vi "Startup.vi"(7 "Application in":refnum<class "Application.lvclass">, 8 "error in (no error)":errorcluster, 11 "Config in":refnum<class "Config.lvclass">) -> (0 "error out":errorcluster, 3 "Config out":refnum<class "Config.lvclass">, 5 "Application out":refnum<class "Application.lvclass">)   [LabVIEW 2019, in "Config.lvclass"]
doc: "Developed by Kevin Thompson\nkevin@thompsonengineering.net\n\nCopyright 2018-2020\nThompson Engineering, LLC"
uses:
  Config.lvclass
  Application/Application.lvclass
  DataTypes/Config Settings.ctl
  Application/DataTypes/Settings--cluster.ctl
  Main/DataTypes/Settings--cluster.ctl
  Main/support/Data Algorithms/subvis/DataTypes/Gain control.ctl
  Main/support/Data Algorithms/subvis/DataTypes/ESR scaling--cluster.ctl
  DAQ_Engine/DataTypes/Settings--cluster.ctl
  Common/DataTypes/Measurement Config--cluster.ctl
  Common/DataTypes/Acquisition Mode--cluster.ctl
  Log_Engine/DataTypes/Settings--cluster.ctl
  Config.lvclass/Config.ctl
  Application/Application.lvclass/Application.ctl
  Accessors/Get Application Settings.vi
  Application/Accessors/Set Settings.vi
  Common/Startup/GBL System.vi
  Log_Engine/Log_Engine.lvclass
  DAQ_Engine/DAQ_Engine.lvclass
  Main/Main.lvclass
  Common/DataTypes/TD GetSet ActionSelect--enum.ctl
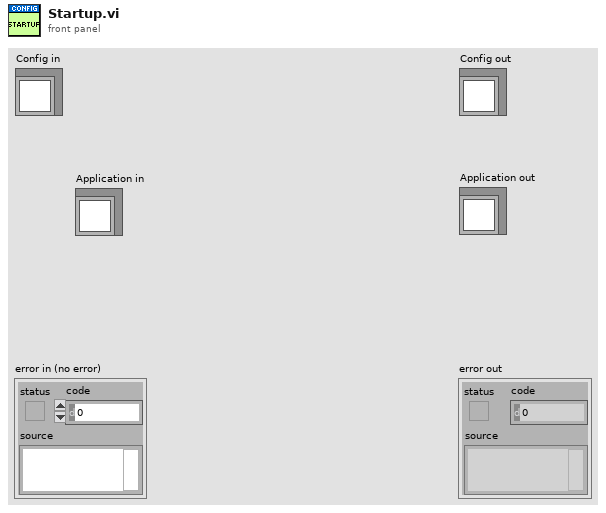
[diagram p1: front panel]
types:
  T1 = typedef "TD GetSet ActionSelect--enum.ctl" = enum16{"Init", "Get", "Set"}
  T2 = typedef "Config.lvclass/Config Settings.ctl" = cluster{"Application Settings":T3, "Main Settings":T4, "DAQ Settings":T7, "LogEngine Settings":T10}
  T3 = typedef "Application.lvclass/Settings--cluster.ctl" = cluster{"Simulation":bool}
  T4 = typedef "Main.lvclass/Settings--cluster.ctl" = cluster{"Simulation":bool, "Signal scaling":T5[], "ESR scaling":T6[], "num readings to average":i32[], "ESR alarm threshhold (%)":i32[], "UseDummyVrms":bool, "Dummy Vrms":dbl, "Inverter Database File":path, "default Inverter (name)":string[]}
  T5 = typedef "Main.lvclass/Gain control.ctl" = cluster{"Iin ripple gain":dbl, "Iout ripple gain":dbl, "Iout 60Hz gain ":dbl, "Vout 60Hz gain ":dbl, "Iin ripple offest":dbl, "Iout ripple offset":dbl, "Iout 60Hz offset":dbl, "Vout 60Hz offset":dbl}
  T6 = typedef "Main.lvclass/ESR scaling--cluster.ctl" = cluster{"Gain":dbl, "Offset":dbl}
  T7 = typedef "DAQ_Engine.lvclass/Settings--cluster.ctl" = cluster{"Simulation":bool, "Initial ErrReporting setting":i32, "Initial Measurement settings":T8, "Acquisition mode":T9, "DemoMode":bool, "RIO Device":string}
  T8 = typedef "Measurement Config--cluster.ctl" = cluster{"Data Rate 9775":dbl, "Data Rate 9215":dbl, "Samples RMS 9215":u32, "Samples RMS 9775":u32}
  T9 = typedef "Acquisition Mode--cluster.ctl" = enum16{"3phase", "Single"}
  T10 = typedef "Log_Engine.lvclass/Settings--cluster.ctl" = cluster{"Simulation":bool, "TDMS_FolderPath":string, "CSV_FolderPath":string, "TDMS_FileName_Prefix":string, "CSV_FileName_Prefix":string, "TDMS_LogDuration(s)":dbl, "CSV_LogDuration(s)":dbl}
  T11 = typedef "TD Pathnames--cluster.ctl" = cluster{"RunTimeSys?":bool, "AppFolder":path, "ExecutablePath":path, "ConfigFolder":path, "DataLogFolder":path, "SystemLogFolder":path, "SeqFolder":path, "MainStartupPathname":path, "MainUIPathname":path, "SystemEventsFile":path, "SeqEventsFile":path, "Config SettingsFile":path, "DAQ IOConfigFile":path, "SystemSimulation":bool}
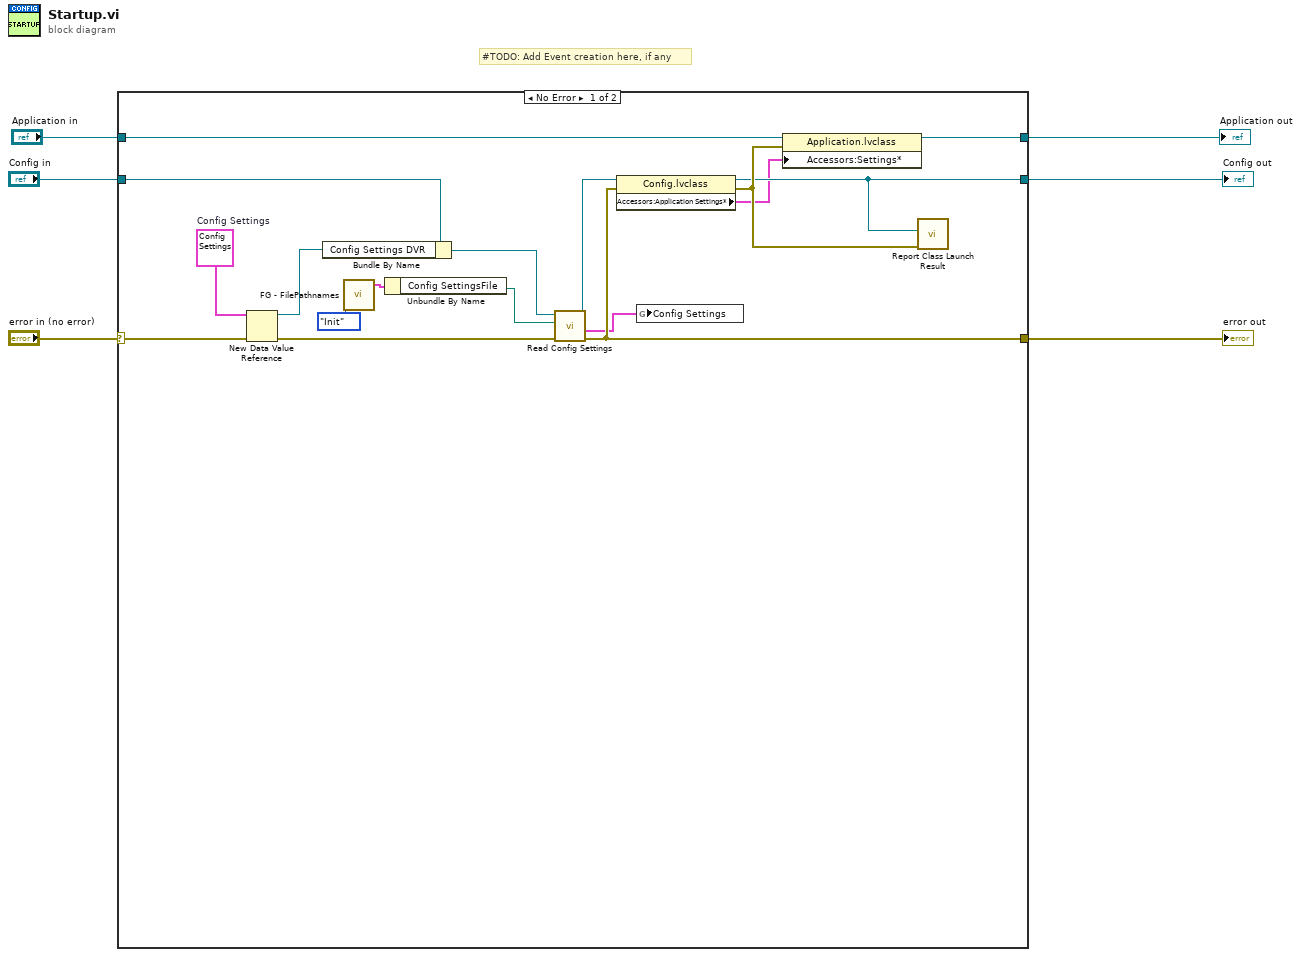
[diagram p0: block diagram]
diagram:
  # "#TODO: Add Event creation here, if any"
  n1 = case shown="No Error" "error in (no error)" {
    selector: "error in (no error)" -> [w23 w26]
    tunnel: [w15 w26] -> w5
    tunnel: [w10 w25] -> w3
    tunnel: "Config in" -> [w21 w25]
    tunnel: "Application in" -> [w14 w24]
    tunnel: [w11 w24] -> w1
    frame No Error {
      w16 = T2 {"Application Settings"={"Simulation"=FALSE}, "Main Settings"={"Simulation"=FALSE, "Signal scaling"=[], "ESR scaling"=[], "num readings to average"=[], "ESR alarm threshhold (%)"=[], "UseDummyVrms"=FALSE, "Dummy Vrms"=0.0, "Inverter Database File"=path "", "default Inverter (name)"=[]}, "DAQ Settings"={"Simulation"=FALSE, "Initial ErrReporting setting"=0, "Initial Measurement settings"={"Data Rate 9775"=3.0, "Data Rate 9215"=1200000.0, "Samples RMS 9215"=480000, "Samples RMS 9775"=3}, "Acquisition mode"=enum."3phase", "DemoMode"=FALSE, "RIO Device"=""}, "LogEngine Settings"={"Simulation"=FALSE, "TDMS_FolderPath"="", "CSV_FolderPath"="", "TDMS_FileName_Prefix"="", "CSV_FileName_Prefix"="", "TDMS_LogDuration(s)"=0.0, "CSV_LogDuration(s)"=0.0}}  # Config Settings
      n2 = New Data Value Reference(data value=w16, error in=w23) -> (data value reference=w22:refnum<data-value>, error out=w20:errorcluster)
      n3 = Bundle By Name(cluster=w21, "Config Settings DVR"=w22) -> (w17:refnum<class "Config.lvclass">)
      n4 = call "FG - FilePathnames.vi"("action (Get)"=TD_GetSet_ActionSelect--enum."Init") -> ("FilePaths out"=w19:T11)  [unwired: 3 in, 1 out]
      n5 = Unbundle By Name(w19) -> ("Config SettingsFile"=w18:path)
      n6 = call "Read Config Settings.vi"("error in (no error)"=w20, "ConfigFile"=w18, "Config in"=w17) -> ("error out"=w15:errorcluster, "Config Settings"=w8:T2, "Config out"=w13:refnum<class "Config.lvclass">)  [unwired: 4 in, 2 out]
      n7 = property class="Config.lvclass"(reference=w13, error in=w15) -> (reference out=w10:refnum<class "Config.lvclass">, error out=w12:errorcluster, "Accessors:Application Settings*"=w9:T3)
      n8 = global write "GBL System.vi" "Config Settings"(w8) -> ()
      n9 = property class="Application.lvclass"(reference=w14, error in=w12, "Accessors:Settings*"=w9) -> (reference out=w11:refnum<class "Application.lvclass">)  [unwired: 1 out]
      n10 = call "Report Class Launch Result.vi"("Object"=w10, "error in (no error)"=w12) -> ()  [unwired: 8 in, 1 out]
    }
    frame Error {
    }
  }
  "error out" <- w5
  "Config out" <- w3
  "Application out" <- w1
